vi "decodeArray.vi"(8 "error in (no error)":errorcluster, 10 "ByteArray":u8[](array[numeric]) format="%.0x") -> (0 "error out":errorcluster, 2 "variant":variant, 3 "ByteArray":u8[](array[numeric]), 5 "Type":string)   [LabVIEW 2020, in "MsgPack.lvlib"]
uses:
  MsgPack.lvlib
  <vilib>/Utility/error.llb/Error Cluster From Error Code.vi
  <vilib>/ErrorRing/Error Ring.xnode
panel:
  out "Array":string[](array[string])
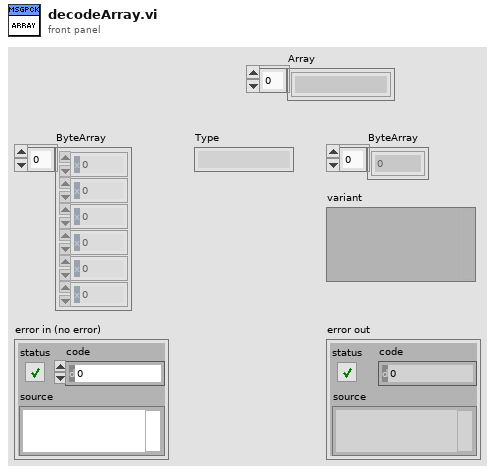
[diagram p1: front panel]
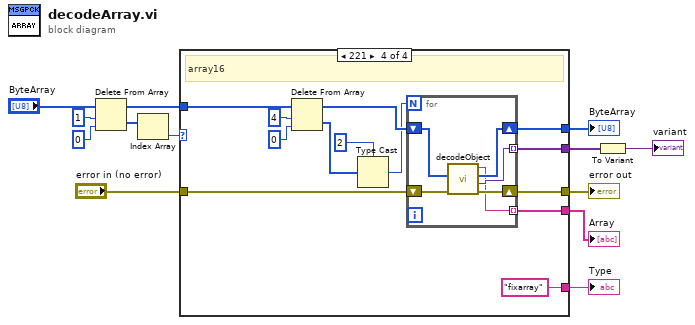
[diagram p0: block diagram]
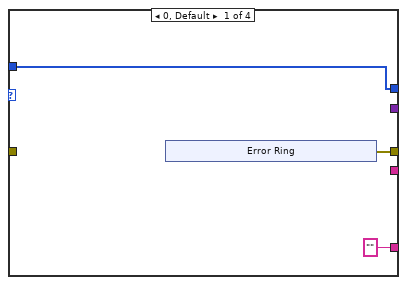
[diagram p2: hidden frame]
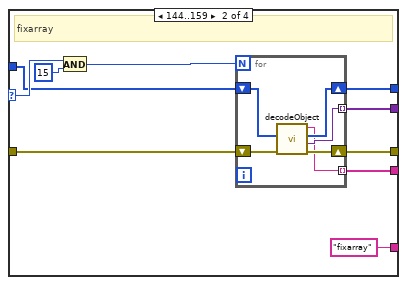
[diagram p3: hidden frame]
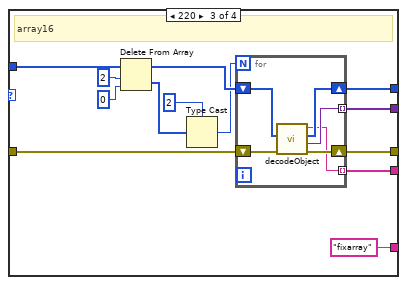
[diagram p4: hidden frame]
diagram:
  n1 = Delete From Array(array="ByteArray", length=1, index=0) -> (deleted portion=w4:u8[], array with subset deleted=w3:u8[])
  n2 = Index Array(array=w4) -> (element=w10:u8)  [unwired: 1 in]
  n3 = case shown="221" w10 {
    selector: w10 -> [_ w30 _ _]
    tunnel: [w16 w25 w48 w67] -> w12
    tunnel: "error in (no error)" -> [_ w26 w49 w68]
    tunnel: ["" "fixarray" "fixarray" "fixarray"] -> w9
    tunnel: [_ w24 w47 w66] -> w8
    tunnel: w3 -> [w14 w27 w45 w64]
    tunnel: [_ w23 w46 w65] -> w7
    tunnel: [w14 w22 w39 w58] -> w2
    frame 0, Default {
      n4 = xnode "Error Ring"() -> ("error out"=w16:errorcluster)
    }
    frame 144..159 {
      # "fixarray"
      n5 = And(x=w30, y=u8 15) -> (x .and. y?=w28:u8)
      n6 = for {
        N: w28 -> [_]
        shift-right: [w34] -> w22
        shift-left: w27 -> [w32]
        tunnel: [w33] -> w23 mode=indexing
        shift-right: [w36] -> w25
        shift-left: w26 -> [w37]
        tunnel: [w35] -> w24 mode=indexing
        n7 = call "decodeObject.vi"("error in (no error)"=w37, "ByteArray"=w32) -> ("error out"=w36:errorcluster, "Variant"=w35:variant, "RemainingBytes"=w34:u8[], "Type"=w33:string)  [unwired: 6 in]
      }
    }
    frame 220 {
      # "array16"
      n8 = Delete From Array(array=w45, length=2, index=0) -> (deleted portion=w42:u8[], array with subset deleted=w43:u8[])
      n9 = Type Cast(type=u16 2 ("length"), x=w42) -> (*(type *) &x=w41:u16)
      n10 = for {
        N: w41 -> [_]
        shift-right: [w53] -> w39
        shift-left: w43 -> [w51]
        tunnel: [w52] -> w46 mode=indexing
        shift-right: [w55] -> w48
        shift-left: w49 -> [w56]
        tunnel: [w54] -> w47 mode=indexing
        n11 = call "decodeObject.vi"("error in (no error)"=w56, "ByteArray"=w51) -> ("error out"=w55:errorcluster, "Variant"=w54:variant, "RemainingBytes"=w53:u8[], "Type"=w52:string)  [unwired: 6 in]
      }
    }
    frame 221 {
      # "array16"
      n12 = Delete From Array(array=w64, length=4, index=0) -> (deleted portion=w61:u8[], array with subset deleted=w62:u8[])
      n13 = Type Cast(type=u32 2 ("length"), x=w61) -> (*(type *) &x=w60:u32)
      n14 = for {
        N: w60 -> [_]
        shift-right: [w72] -> w58
        shift-left: w62 -> [w70]
        tunnel: [w71] -> w65 mode=indexing
        shift-right: [w74] -> w67
        shift-left: w68 -> [w75]
        tunnel: [w73] -> w66 mode=indexing
        n15 = call "decodeObject.vi"("error in (no error)"=w75, "ByteArray"=w70) -> ("error out"=w74:errorcluster, "Variant"=w73:variant, "RemainingBytes"=w72:u8[], "Type"=w71:string)  [unwired: 6 in]
      }
    }
  }
  "error out" <- w12
  "Type" <- w9
  "Array" <- w7
  "ByteArray" <- w2
  n16 = To Variant(anything=w8) -> (Variant=→"variant":variant)
